vi "addError.vi"(7 "execution time (sec)":dbl, 8 "error in (no error)":errorcluster, 9 "test error":errorcluster, 10 "test":refnum<class>, 11 "TestResult in":refnum<class "TestResult.lvclass">) -> (0 "error out":errorcluster, 3 "TestResult out":refnum<class "TestResult.lvclass">)   [LabVIEW 2019, in "TestResult.lvclass"]
uses:
  TestResult.lvclass
  resultStatusChanged--Cluster.ctl
  resultStatus--enum.ctl
  TestResult.lvclass/TestResult.ctl
panel:
  # "JKI VI Tester for LabVIEW\nhttp://jkisoft.com/vi-tester\nCopyright (C) 2007-2009, JKI <info@jkisoft.com>\nALL RIGHTS RESERVED"
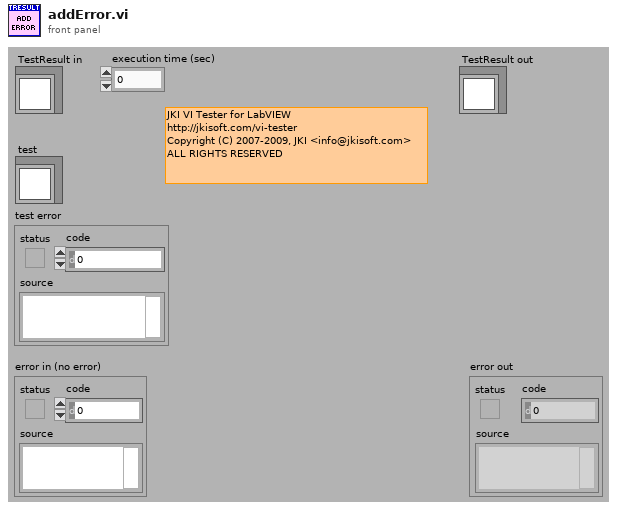
[diagram p1: front panel]
types:
  T1 = typedef "TestResult.lvclass/resultStatusChanged--Cluster.ctl" = cluster{"test":refnum<class>, "resultStatus":T2, "TestResult":refnum<class>, "test error":errorcluster, "execution time (sec)":dbl}
  T2 = typedef "TestResult.lvclass/resultStatus--enum.ctl" = enum16{"testPass", "testFailure", "testError", "testSkipped"}
  T3 = typedef "TestResult.lvclass/errors.ctl" = T4[]
  T4 = typedef "TestResult.lvclass/error.ctl" = cluster{"test":refnum<class>, "error":errorcluster}
  T5 = cluster{"test":refnum<class>, "error IO":errorcluster}
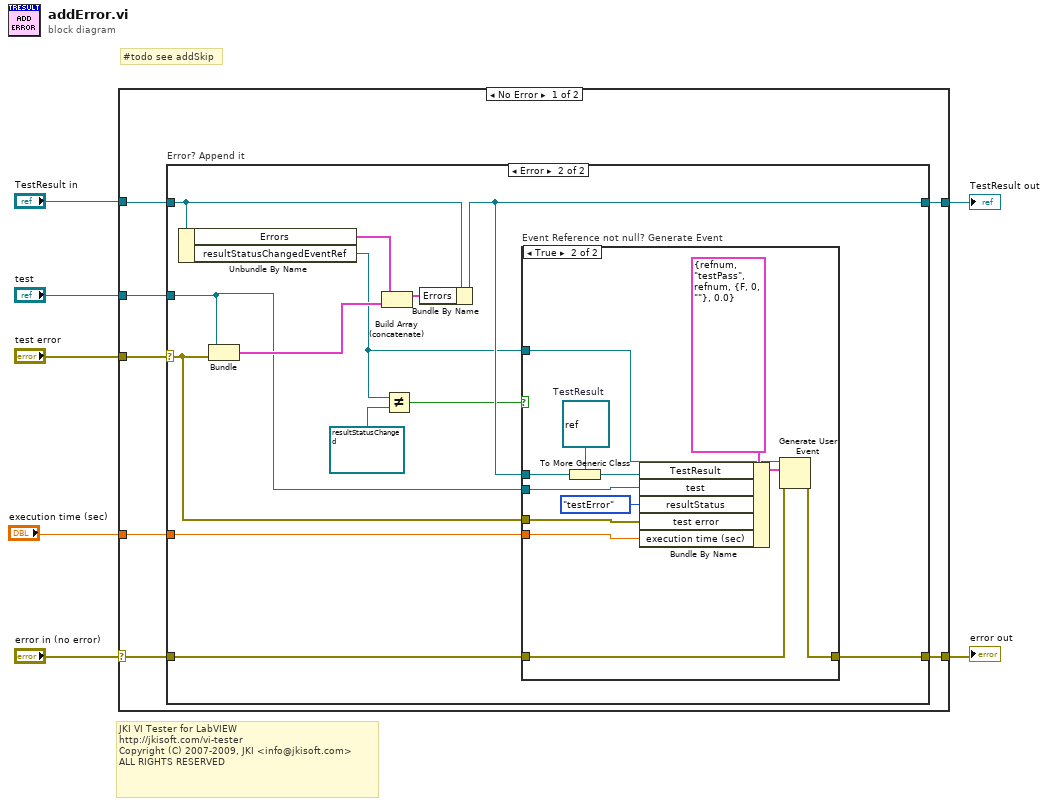
[diagram p0: block diagram]
diagram:
  # "#todo see addSkip"
  # "JKI VI Tester for LabVIEW\nhttp://jkisoft.com/vi-tester\nCopyright (C) 2007-2009, JKI <info@jkisoft.com>\nALL RIGHTS RESERVED"
  n1 = case shown="No Error" "error in (no error)" {
    selector: "error in (no error)" -> [w9 w44]
    tunnel: [w10 w44] -> w6
    tunnel: [w13 w43] -> w4
    tunnel: "TestResult in" -> [w14 w43]
    tunnel: "test" -> [w12 _]
    tunnel: "test error" -> [w11 _]
    tunnel: "execution time (sec)" -> [w8 _]
    frame No Error {
      n2 = case "Error? Append it" shown="Error" w11 {
        selector: w11 -> [w15 w23]
        tunnel: w14 -> [w16 w28]
        tunnel: [w16 w24] -> w13
        tunnel: w12 -> [_ w25]
        tunnel: [w15 w20] -> w10
        tunnel: w9 -> [_ w19]
        tunnel: w8 -> [_ w17]
        frame No Error {
        }
        frame Error {
          n3 = Unbundle By Name(w28) -> ("Errors"=w29:T3, "resultStatusChangedEventRef"=w21:refnum<user-event>)
          n4 = Bundle("test"=w25, "error IO"=w23) -> (w26:T5)  [unwired: 1 in]
          n5 = Build Array (concatenate)(w29, w26) -> (w27:T3)
          n6 = Not Equal?(x=w21, y=refnum<user-event> refnum ("resultStatusChangedEventRef")) -> (x != y?=w18:bool)
          n7 = Bundle By Name(cluster=w28, "Errors"=w27) -> (w24:refnum<class "TestResult.lvclass">)
          n8 = case "Event Reference not null? Generate Event" shown="True" w18 {
            tunnel: w25 -> [_ w41]
            tunnel: w24 -> [_ w39]
            tunnel: w23 -> [_ w37]
            tunnel: w21 -> [_ w36]
            tunnel: [w30 w35] -> w20
            tunnel: w19 -> [w30 w34]
            tunnel: w17 -> [_ w31]
            frame False {
            }
            frame True {
              w32 = refnum<class> refnum  # TestResult
              n9 = To More Generic Class(target class=w32, reference=w39) -> (generic class reference=w33:refnum<class>)
              n10 = Bundle By Name(cluster=T1 {"test"=refnum, "resultStatus"=enum."testPass", "TestResult"=refnum, "test error"={"status"=FALSE, "code"=0, "source"=""}, "execution time (sec)"=0.0} ("event data"), "TestResult"=w33, "test"=w41, "resultStatus"=resultStatus--enum."testError", "test error"=w37, "execution time (sec)"=w31) -> (w40:T1)
              n11 = Generate User Event(user event=w36, event data cluster=w40, error in=w34) -> (error out=w35:errorcluster)  [unwired: 1 in, 1 out]
            }
          }
        }
      }
    }
    frame Error {
    }
  }
  "error out" <- w6
  "TestResult out" <- w4
